vi "frame_scan_addition.vi"(6 "frame scanning?":bool, 8 "amplitude":u16, 9 "scan points cluster in":T1, 10 "y-resolution":u16, 11 "x-resolution":u16) -> (1 "scan points cluster out":T1, 3 "new pixel update?":bool)   [LabVIEW 2010]
uses:
  scan_points_cluster.ctl
  <vilib>/rvi/DataTransferAndStorage/Container/XNode/niFpgaContainer.xnode
  <vilib>/eio/EIONode/EIONode.xnode
  <vilib>/rvi/eio/nirviEIOImplementation/nirviEIOImplementation.xnode
  <vilib>/rvi/eio/common/nirviEmuClasses.ctl
  <vilib>/rvi/FIFO/Fifo_Resource/nirvififoEmulationSetSize.vi
  <vilib>/rvi/DataTransferAndStorage/Container/Common/niFpgaContainerGetUniqueNameForEmu.vi
  <vilib>/rvi/eio/common/nirviEmuTemplateMethod_noerrors.vi
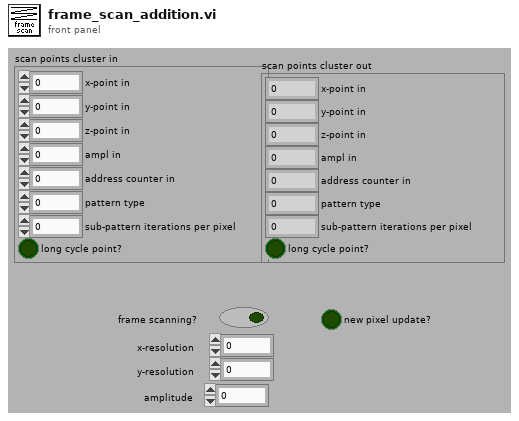
[diagram p1: front panel]
types:
  T1 = typedef "scan_points_cluster.ctl" = cluster{"x-point in":u16, "y-point in":u16, "z-point in":u16, "ampl in":u16, "address counter in":i32, "pattern type":i8, "sub-pattern iterations per pixel":u16, "long cycle point?":bool}
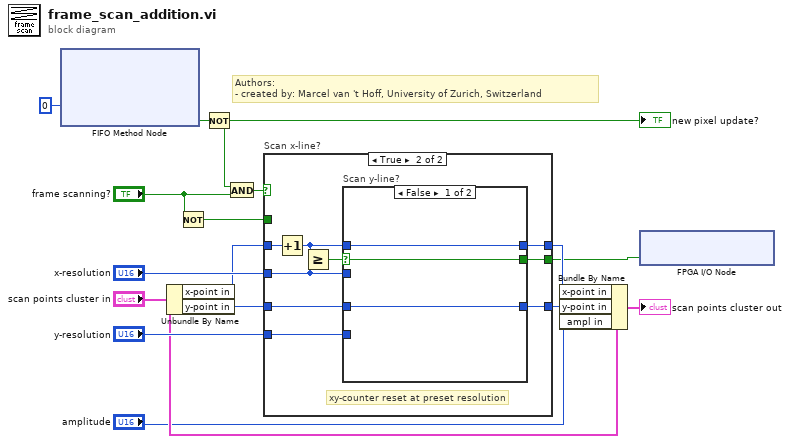
[diagram p0: block diagram]
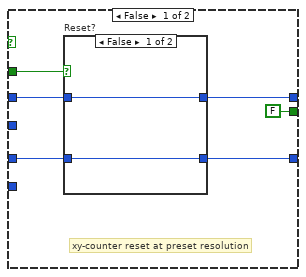
[diagram p2: hidden frame]
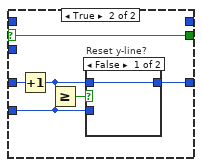
[diagram p4: hidden frame]
diagram:
  # "Authors: \n- created by: Marcel van 't Hoff, University of Zurich, Switzerland"
  n1 = xnode ("FIFO Method Node")("Timeout"=0) -> ("Timed Out?"=w13:bool)  [unwired: 1 in, 2 out]
  n2 = Unbundle By Name("scan points cluster in") -> ("x-point in"=w8:u16, "y-point in"=w7:u16)
  n3 = Not(x="frame scanning?") -> (.not. x?=w9:bool)
  n4 = Not(x=w13) -> (.not. x?=w12:bool)
  "new pixel update?" <- w12
  n5 = And(x=w12, y="frame scanning?") -> (x .and. y?=w11:bool)
  n6 = case "Scan x-line?" shown="True" w11 {
    tunnel: "x-resolution" -> [_ w30]
    tunnel: w8 -> [w20 w33]
    tunnel: w7 -> [w18 w28]
    tunnel: "y-resolution" -> [_ w27]
    tunnel: [w21 w31] -> w6
    tunnel: [w19 w26] -> w4
    tunnel: w9 -> [w22 _]
    tunnel: [FALSE w25] -> w1
    frame False {
      # "xy-counter reset at preset resolution"
      n7 = case "Reset?" shown="False" w22 {
        tunnel: [w24 _] -> w21
        tunnel: w20 -> [w24 _]
        tunnel: [w23 _] -> w19
        tunnel: w18 -> [w23 _]
        frame False {
        }
        frame True {
        }
      }
    }
    frame True {
      # "xy-counter reset at preset resolution"
      n8 = Increment(x=w33) -> (x+1=w29:u16)
      n9 = Greater Or Equal?(x=w29, y=w30) -> (x >= y?=w32:bool)
      n10 = case "Scan y-line?" shown="False" w32 {
        selector: w32 -> [w34 w37]
        tunnel: [w36 _] -> w31
        tunnel: w30 -> [_ _]
        tunnel: w29 -> [w36 _]
        tunnel: w28 -> [w35 w42]
        tunnel: w27 -> [_ w38]
        tunnel: [w35 w39] -> w26
        tunnel: [w34 w37] -> w25
        frame False {
        }
        frame True {
          n11 = Increment(x=w42) -> (x+1=w40:u16)
          n12 = Greater Or Equal?(x=w40, y=w38) -> (x >= y?=w41:bool)
          n13 = case "Reset y-line?" shown="False" w41 {
            tunnel: w40 -> [w43 _]
            tunnel: [w43 _] -> w39
            tunnel: w38 -> [_ _]
            frame False {
            }
            frame True {
            }
          }
        }
      }
    }
  }
  n14 = Bundle By Name(cluster="scan points cluster in", "x-point in"=w6, "y-point in"=w4, "ampl in"="amplitude") -> (→"scan points cluster out":T1)
  n15 = xnode "FPGA I/O Node"("Connector0/DIO32"=w1) -> ()  [unwired: 1 in, 1 out]
